vi "Find by ID.vi"(8 "error in (no error)":errorcluster, 11 "Entity Repository in":refnum<class "Entity Repository.lvclass">) -> (0 "error out":errorcluster, 3 "Entity Repository out":refnum<class "Entity Repository.lvclass">)   [LabVIEW 2020, in "Conditu2.lvlib" / "Entity Repository.lvclass"]
uses:
  Entity Repository.lvclass
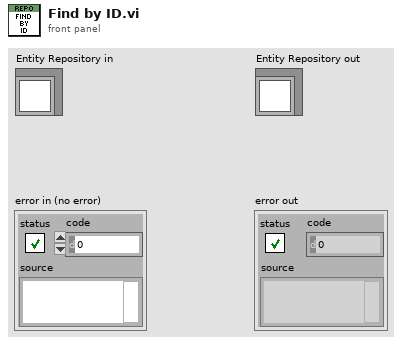
[diagram p1: front panel]
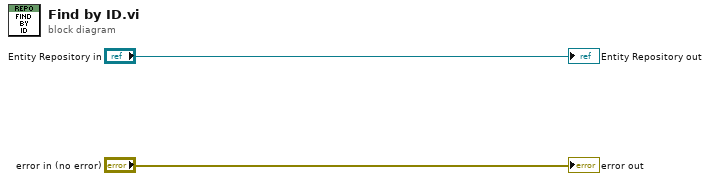
[diagram p0: block diagram]
diagram:
  "error out" <- "error in (no error)"
  "Entity Repository out" <- "Entity Repository in"
